vi "request.has params.vi"(8 "error in (no error)":errorcluster, 11 "Request in":refnum<class "Request.lvclass">) -> (0 "error out":errorcluster, 2 "has params?":bool, 3 "Request out":refnum<class "Request.lvclass">)   [LabVIEW 2017, in "Request.lvclass"]
uses:
  Request.lvclass
  <vilib>/Utility/Data Type/Type Definitions/Data Type.ctl
  Request.lvclass/Request.ctl
  params/params.lvclass
  <vilib>/Utility/Data Type/NI_Data Type.lvlib
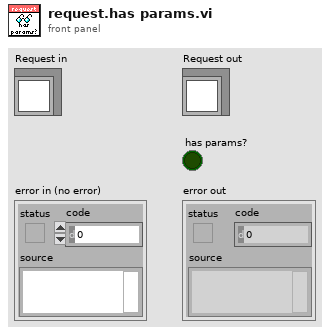
[diagram p1: front panel]
types:
  T1 = typedef "NI_Data Type.lvlib/Data Type.ctl" = enum8{"Invalid Type", "Void", "I8", "I16", "I32", "I64", "U8", "U16", "U32", "U64", "Single Float", "Double Float", "Extended Float", "Single Complex", "Double Complex", "Extended Complex", "Enum U8", "Enum U16", "Enum U32", "Enum U64", "Single Float With Unit", "Double Float With Unit", "Extended Float With Unit", "Single Complex with Unit", "Double Complex with Unit", "Extended Complex with Unit", "Boolean", "String", "Path", "Picture", "Tag", "Array", "Cluster", "Variant", "LV Variant", "Waveform", "Timestamp", "Digital Waveform", "Digital Data", "ExpressData", "Refnum", "External Data", "VI", "Poly VI", "LabVIEW Class Instance", "Fixed Point"}
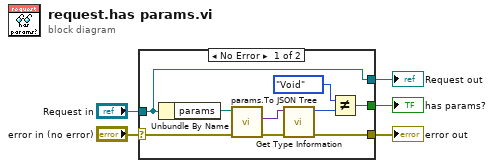
[diagram p0: block diagram]
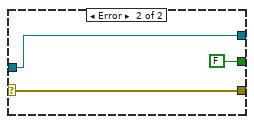
[diagram p2: hidden frame]
diagram:
  n1 = case shown="No Error" "error in (no error)" {
    selector: "error in (no error)" -> [w11 w17]
    tunnel: [w9 w17] -> w4
    tunnel: [w14 w16] -> w2
    tunnel: "Request in" -> [w14 w16]
    tunnel: [w13 FALSE] -> w1
    frame No Error {
      n2 = Unbundle By Name(w14) -> ("params"=w12:refnum<class "params.lvclass">)
      n3 = call "params.To JSON Tree.vi"("error in (no error)"=w11, "params in"=w12) -> ("error out"=w10:errorcluster, "JSON Value out"=w6:variant)  [unwired: 7 in, 1 out]
      n4 = call <vilib>:"Get Type Information.vi"("error in (no error)"=w10, "Variant"=w6) -> ("error out"=w9:errorcluster, "Type"=w8:T1)  [unwired: 5 in, 3 out]
      n5 = Not Equal?(x=Data_Type."Void", y=w8) -> (x != y?=w13:bool)
    }
    frame Error {
    }
  }
  "error out" <- w4
  "Request out" <- w2
  "has params?" <- w1
